vi "Initialize Channels.vi"(8 "error in":errorcluster, 11 "PowerSupply in":refnum<class "PowerSupply.lvclass">) -> (0 "error out":errorcluster, 3 "PowerSupply out":refnum<class "PowerSupply.lvclass">)   [LabVIEW 2019, in "PowerSupply.lvlib" / "PowerSupply.lvclass"]
uses:
  Library/PowerSupply.lvclass
  Library/PowerSupply.lvclass/PowerSupply.ctl
  Custom Controls/Settings.ctl
  Custom Controls/Sense Point.ctl
  Custom Controls/OCP Mode.ctl
  Custom Controls/Limits.ctl
  Custom Controls/Status_Flags.ctl
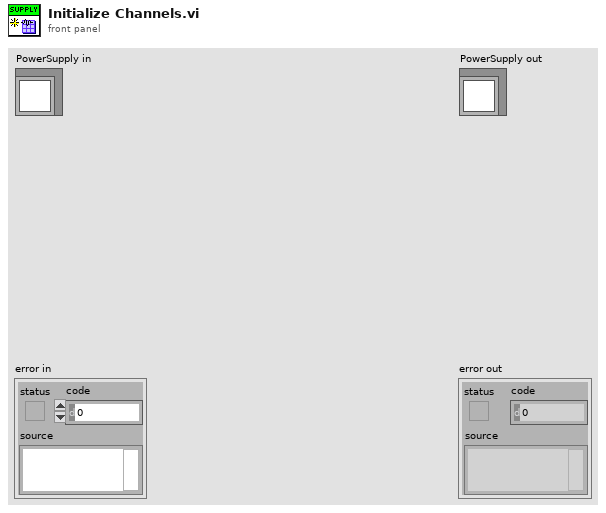
[diagram p1: front panel]
types:
  T1 = typedef "PowerSupply.lvlib/PowerSupply.lvclass/Status_Flags.ctl" = cluster{"Interlock":bool, "OVP":bool, "OCP":bool, "Output":bool}
  T2 = typedef "PowerSupply.lvlib/PowerSupply.lvclass/Limits.ctl" = cluster{"Max_Current":dbl, "Max_Voltage":dbl, "Max_Current_Ramp":dbl, "Max_Voltage_Ramp":dbl, "Max_OCP":dbl, "Max_OVP":dbl}
  T3 = typedef "PowerSupply.lvlib/PowerSupply.lvclass/Settings.ctl" = cluster{"Voltage":dbl, "Current":dbl, "Output":bool, "OverVolt_Protect":dbl, "OverCurrent_Protect":dbl, "OVP":bool, "OCP":bool, "Interlock":bool, "Volt_Ramp":dbl, "Current_Ramp":dbl, "Sense Point":T4, "OCP Mode":T5, "Sharing":bool}
  T4 = typedef "PowerSupply.lvlib/PowerSupply.lvclass/Sense Point.ctl" = enum16{"Local", "Remote"}
  T5 = typedef "PowerSupply.lvlib/PowerSupply.lvclass/OCP Mode.ctl" = enum16{"Shutdown", "Foldback"}
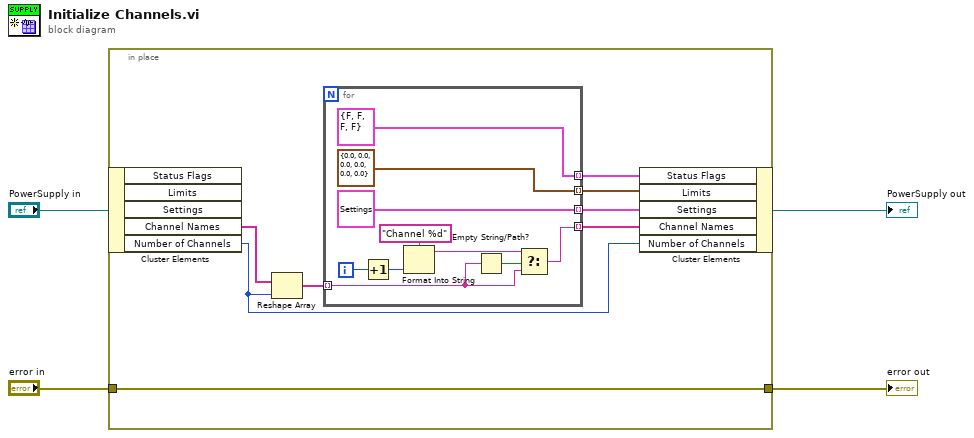
[diagram p0: block diagram]
diagram:
  n1 = in-place {
    in-place-border: "error in" -> [w11]
    in-place-border: [w11] -> w1
    n2 = in-place-cluster #1("PowerSupply in") -> ("Channel Names"=w9:string[], "Number of Channels"=w7:i32)  [unwired: 3 out]
    n3 = Reshape Array(w9, w7) -> (w10:string[])
    n4 = for {
      tunnel: [w20] -> w12 mode=indexing
      tunnel: w10 -> [w21] mode=indexing
      tunnel: [T3 {"Voltage"=0.0, "Current"=0.0, "Output"=FALSE, "OverVolt_Protect"=0.0, "OverCurrent_Protect"=0.0, "OVP"=FALSE, "OCP"=FALSE, "Interlock"=FALSE, "Volt_Ramp"=0.0, "Current_Ramp"=0.0, "Sense Point"=enum."Local", "OCP Mode"=enum."Shutdown", "Sharing"=FALSE} ("Settings")] -> w8 mode=indexing
      tunnel: [T2 {"Max_Current"=0.0, "Max_Voltage"=0.0, "Max_Current_Ramp"=0.0, "Max_Voltage_Ramp"=0.0, "Max_OCP"=0.0, "Max_OVP"=0.0} ("Limits")] -> w6 mode=indexing
      tunnel: [T1 {"Interlock"=FALSE, "OVP"=FALSE, "OCP"=FALSE, "Output"=FALSE} ("Status")] -> w5 mode=indexing
      i -> [w18]
      n5 = Increment(x=w18) -> (x+1=w17:i32)
      n6 = Format Into String(format string="Channel %d", w17) -> (resulting string=w16:string)  [unwired: 2 in, 1 out]
      n7 = Empty String/Path?(string/path=w21) -> (empty?=w22:bool)
      n8 = Select(t=w16, s=w22, f=w21) -> (s? t:f=w20:string)
    }
    n9 = in-place-cluster #1("Status Flags"=w5, "Limits"=w6, "Settings"=w8, "Channel Names"=w12, "Number of Channels"=w7) -> (→"PowerSupply out":refnum<class "PowerSupply.lvclass">)
  }
  "error out" <- w1
